vi "Power Output Display Key Array.vi"(4 "Conversion":enum16{"Cluster - HTML", "HTML - Cluster"}(ring), 6 "Display Key Array In":T2, 7 "Display Cluster In":T1={"Frequency"={"Min"=-160.0, "Max"=-60.0}, "Power"={"Min"=0, "Max"=0}}) -> (1 "Display Cluster Out":T1={"Frequency"={"Min"=-160.0, "Max"=-60.0}, "Power"={"Min"=0, "Max"=0}}, 2 "Display HTML Out":string)   [LabVIEW 2011]
uses:
  ITK EXT/utils/keyedarr.llb/Keyed Array.ctl
  TypeDefs/Power Output Display Parameters.ctl
  ITK EXT/utils/strutil.llb/Case Matching.ctl
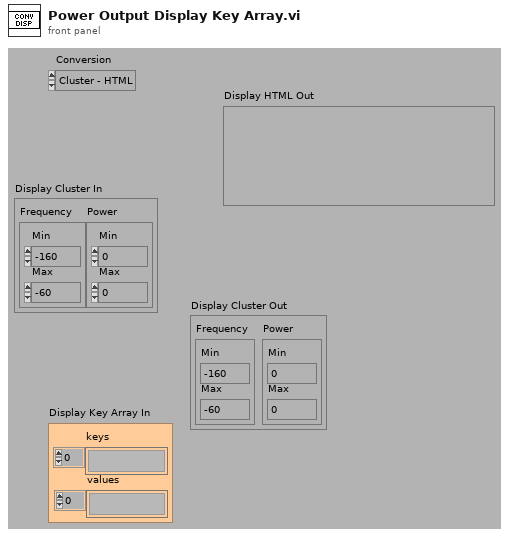
[diagram p1: front panel]
types:
  T1 = typedef "Power Output Display Parameters.ctl" = cluster{"Frequency":cluster{"Min":dbl, "Max":dbl}, "Power":cluster{"Min":i32, "Max":i32}}
  T2 = typedef "Keyed Array.ctl" = cluster{"keys":string[], "values":string[]}
  T3 = typedef "Case Matching.ctl" = enum16{"a != A", "a == A", "system"}
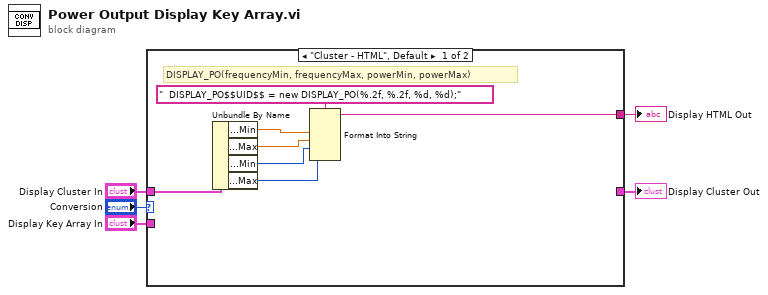
[diagram p0: block diagram]
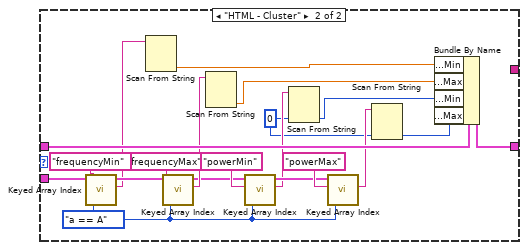
[diagram p2: hidden frame]
diagram:
  n1 = case shown="\"Cluster - HTML\", Default" "Conversion" {
    tunnel: "Display Key Array In" -> [_ w15]
    tunnel: "Display Cluster In" -> [w12 w32]
    tunnel: [w7 _] -> w3
    tunnel: [_ w31] -> w2
    frame "Cluster - HTML", Default {
      # "DISPLAY_PO(frequencyMin, frequencyMax, powerMin, powerMax)"
      n2 = Unbundle By Name(w12) -> ("Frequency.Min"=w10:dbl, "Frequency.Max"=w9:dbl, "Power.Min"=w8:i32, "Power.Max"=w6:i32)
      n3 = Format Into String(format string="  DISPLAY_PO$$UID$$ = new DISPLAY_PO(%.2f, %.2f, %d, %d);", w10, w9, w8, w6) -> (resulting string=w7:string)  [unwired: 2 in, 1 out]
    }
    frame "HTML - Cluster" {
      w13 = 0 ("Measure.Ref Units")
      w14 = Case_Matching."a == A" ("case matching (sensitive)")
      n4 = call "Keyed Array Index.vi"("case matching (sensitive)"=w14, "key"="frequencyMin", "array in"=w15) -> ("value"=w24:string, "duplicate array"=w28:T2)  [unwired: 1 in, 2 out]
      n5 = Scan From String(input string=w24) -> (output 1=w25:dbl)  [unwired: 3 in, 4 out]
      n6 = call "Keyed Array Index.vi"("case matching (sensitive)"=w14, "key"="frequencyMax", "array in"=w28) -> ("value"=w23:string, "duplicate array"=w21:T2)  [unwired: 1 in, 2 out]
      n7 = Scan From String(input string=w23) -> (output 1=w22:dbl)  [unwired: 3 in, 4 out]
      n8 = call "Keyed Array Index.vi"("case matching (sensitive)"=w14, "key"="powerMin", "array in"=w21) -> ("value"=w19:string, "duplicate array"=w20:T2)  [unwired: 1 in, 2 out]
      n9 = Scan From String(input string=w19, default 1=w13) -> (output 1=w18:i32)  [unwired: 3 in, 3 out]
      n10 = call "Keyed Array Index.vi"("case matching (sensitive)"=w14, "key"="powerMax", "array in"=w20) -> ("value"=w17:string)  [unwired: 1 in, 3 out]
      n11 = Scan From String(input string=w17, default 1=w13) -> (output 1=w16:i32)  [unwired: 3 in, 3 out]
      n12 = Bundle By Name(cluster=w32, "Frequency.Min"=w25, "Frequency.Max"=w22, "Power.Min"=w18, "Power.Max"=w16) -> (w31:T1)
    }
  }
  "Display HTML Out" <- w3
  "Display Cluster Out" <- w2
